vi "Assert Error Message Contains String.vi"(5 "Expected":string, 7 "Message (\"\")":string, 8 "error in (no error)":errorcluster) -> (0 "error out":errorcluster)   [LabVIEW 2017, in "Transparent Assertions.lvlib" / "Assertions.lvlib"]
doc: "Asserts that the error message of <B>error in</B> matches the expected message. Returns an error if the assertion fails, and optionally appends a custom message to the error."
uses:
  Assertions.lvlib
  Constraints/ErrorMessageContains/ErrorMessageContains.lvclass
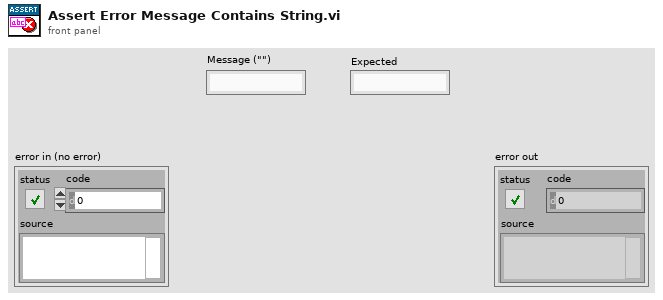
[diagram p1: front panel]
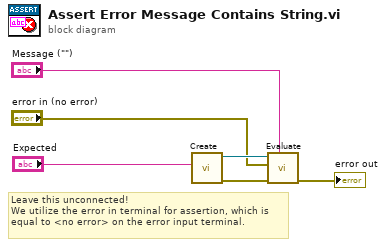
[diagram p0: block diagram]
diagram:
  # "Leave this unconnected!\nWe utilize the error in terminal for assertion, which is\nequal to <no error> on the error input terminal."
  n1 = call "Create.vi"("Expected"="Expected") -> ("error out"=w4:errorcluster, "ErrorMessageContains"=w6:refnum<class "ErrorMessageContains.lvclass">)  [unwired: 9 in]
  n2 = call-dynamic "Evaluate.vi"("Message (\"\")"="Message (\"\")", "error in (no error)"=w4, "Actual"="error in (no error)", "Constraint in"=w6) -> ("error out"=→"error out":errorcluster)  [unwired: 6 in, 1 out]
